vi "CD Init_Prepare Inline Data_Fill Frame Descriptors from BC configuration.vi"(8 "error in (no error)":errorcluster, 11 "RT Channel In":T1 {"RTs"."Mode Codes"."param item refs" format="%.0x"; "RTs"."Mode Codes"."param block data refs"."Data Reference" format="%.0x"; "RTs"."Mode Codes"."Timestamp Channel Data Reference" format="%.0x"; "RTs"."subAddresses"."param item refs" format="%.0x"; "RTs"."subAddresses"."param blocj data refs"."Data Reference" format="%.0x"; "RTs"."subAddresses"."Timestamp Channel Data Reference" format="%.0x"; "RTs"."Status Channel Data Reference" format="%.0x"; "RTs"."Command Channels Refs" format="%.0x"; "BC"."Acyclic Frames Trigger Channels Refs" format="%.0x"; "BC"."Command Channels Refs" format="%.0x"; "BC"."messages"."Timestamp Channel Data Reference" format="%.0x"; "BC"."messages"."Status Channel Data Refs" format="%.0x"; "BC"."messages"."param item refs" format="%.0x"; "BC"."messages"."param Block Data Refs"."Data Reference" format="%.0x"}) -> (0 "error out":errorcluster, 2 "RTs":T13[](array[typedef]) {"Mode Codes"."param item refs" format="%.0x"; "Mode Codes"."param block data refs"."Data Reference" format="%.0x"; "Mode Codes"."Timestamp Channel Data Reference" format="%.0x"; "subAddresses"."param item refs" format="%.0x"; "subAddresses"."param blocj data refs"."Data Reference" format="%.0x"; "subAddresses"."Timestamp Channel Data Reference" format="%.0x"; "Status Channel Data Reference" format="%.0x"; "Command Channels Refs" format="%.0x"}, 3 "Frames Descriptors Out":T18[](array[typedef]) {"RT"."Status Channel Ref" format="%.0x"; "RT"."Words Block Data Refs"."Data Reference" format="%.0x"; "RT"."Timestamp Channel Data Reference" format="%.0x"; "BC"."Status Channel Refs" format="%.0x"; "BC"."param block data refs"."Data Reference" format="%.0x"; "BC"."Timestamp Channel Data Reference" format="%.0x"})   [LabVIEW 2020, in "Ballard MIL-1553 Engine.lvlib"]
uses:
  Ballard MIL-1553 Engine.lvlib
  Controls/RT Inline Frame Descriptor.ctl
  Controls/RT Inline Frame Descriptor_BC.ctl
  <vilib>/NI VeriStand/Custom Device API/Data Reference.ctl
  <vilib>/NI VeriStand/Custom Device API/Block Data Reference.ctl
  <vilib>/NI VeriStand/Custom Device API/Custom Device Item Ref.ctl
  Shared/EncodeDecode/_typedefs/parameter_config_type.ctl
  Shared/EncodeDecode/_typedefs/parameter_config_type_type.ctl
  Shared/EncodeDecode/_typedefs/parameter_config_encoding_type.ctl
  Controls/RT Inline Frame Descriptor_RT.ctl
  Shared/Controls and Global/RT CWD2.ctl
  Shared/Controls and Global/RT CWD1.ctl
  Shared/Controls and Global/RT messageType.ctl
  Shared/Controls and Global/RT Remote Terminal.ctl
  Shared/Controls and Global/RT Remote Terminal_rtMode.ctl
  Shared/Controls and Global/RT Remote Terminal_RT subAddress.ctl
  Shared/Controls and Global/RT Remote Terminal_RT direction.ctl
  Shared/Controls and Global/RT Remote Terminal_RT Mode Code.ctl
  Shared/Controls and Global/RT Channel.ctl
  Shared/Controls and Global/RT BC.ctl
  Shared/Controls and Global/RT Message.ctl
  Shared/Ballard 1553 Shared.lvlib
  <vilib>/NI VeriStand/Custom Device API/Custom Device API.lvlib
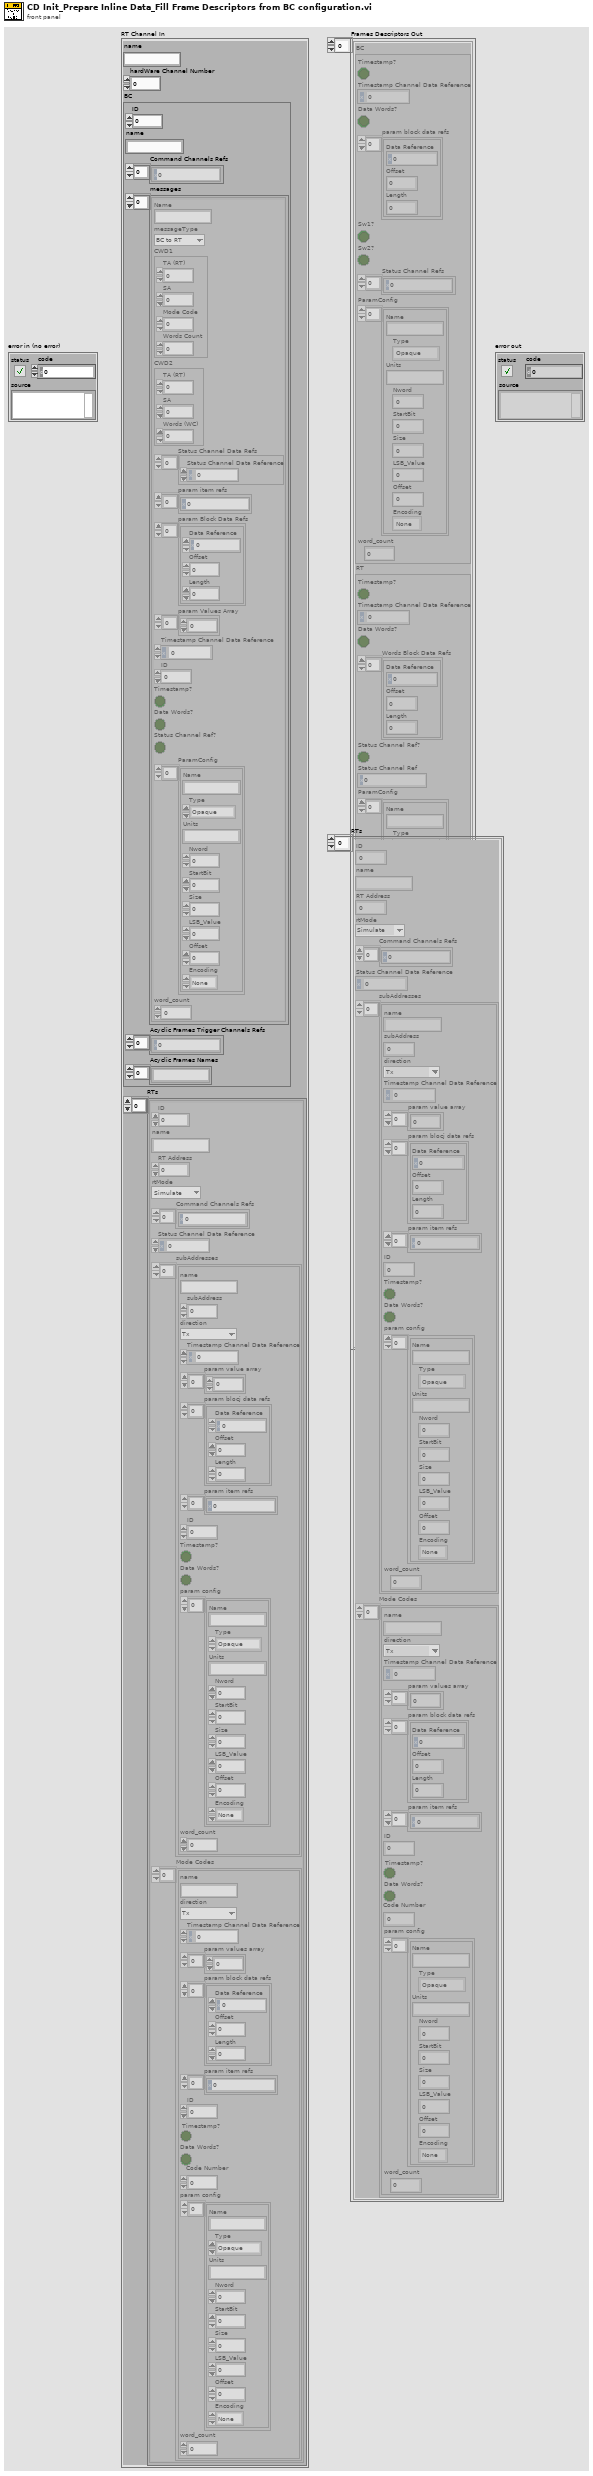
[diagram p1: front panel]
types:
  T1 = typedef "Ballard 1553 Shared.lvlib/RT Channel.ctl" = cluster{"name":string, "hardWare Channel Number":u16, "BC":T2, "RTs":T13[]}
  T2 = typedef "Ballard 1553 Shared.lvlib/RT BC.ctl" = cluster{"ID":i32, "name":string, "Command Channels Refs":T3[], "messages":T4[], "Acyclic Frames Trigger Channels Refs":T3[], "Acyclic Frames Names":string[]}
  T3 = typedef "Custom Device API.lvlib/Custom Device Item Ref.ctl" = u64
  T4 = typedef "Ballard 1553 Shared.lvlib/RT Message.ctl" = cluster{"Name":string, "messageType":T5, "CWD1":T6, "CWD2":T7, "Status Channel Data Refs":T8[], "param item refs":T3[], "param Block Data Refs":T9[], "param Values Array":u16[], "Timestamp Channel Data Reference":T8, "ID":i32, "Timestamp?":bool, "Data Words?":bool, "Status Channel Ref?":bool, "ParamConfig":T10[], "word_count":u8}
  T5 = typedef "Ballard 1553 Shared.lvlib/RT messageType.ctl" = enum16{"BC to RT", "RT to BC", "RT to RT", "MC (Rx)", "MC (Tx)"}
  T6 = typedef "Ballard 1553 Shared.lvlib/RT CWD1.ctl" = cluster{"TA (RT)":i8, "SA":i8, "Mode Code":i8, "Words Count":i8}
  T7 = typedef "Ballard 1553 Shared.lvlib/RT CWD2.ctl" = cluster{"TA (RT)":i8, "SA":i8, "Words (WC)":i8}
  T8 = typedef "Custom Device API.lvlib/Data Reference.ctl" = i32
  T9 = typedef "Custom Device API.lvlib/Block Data Reference.ctl" = cluster{"Data Reference":T8, "Offset":u64, "Length":u64}
  T10 = typedef "parameter_config_type.ctl" = cluster{"Name":string, "Type":T11, "Units":string, "Nword":i32, "StartBit":i32, "Size":i32, "LSB_Value":i32, "Offset":i32, "Encoding":T12}
  T11 = typedef "parameter_config_type_type.ctl" = enum16{"Opaque", "Enum", "Float", "Integer", "Bcd", "Bool"}
  T12 = typedef "parameter_config_encoding_type.ctl" = enum16{"None", "2-complement", "Unsigned"}
  T13 = typedef "Ballard 1553 Shared.lvlib/RT Remote Terminal.ctl" = cluster{"ID":i32, "name":string, "RT Address":i32, "rtMode":T14, "Command Channels Refs":T3[], "Status Channel Data Reference":T8, "subAddresses":T15[], "Mode Codes":T17[]}
  T14 = typedef "Ballard 1553 Shared.lvlib/RT Remote Terminal_rtMode.ctl" = enum16{"Simulate", "Monitor", "Disable"}
  T15 = typedef "Ballard 1553 Shared.lvlib/RT Remote Terminal_RT subAddress.ctl" = cluster{"name":string, "subAddress":i8, "direction":T16, "Timestamp Channel Data Reference":T8, "param value array":u16[], "param blocj data refs":T9[], "param item refs":T3[], "ID":i32, "Timestamp?":bool, "Data Words?":bool, "param config":T10[], "word_count":u8}
  T16 = typedef "Ballard 1553 Shared.lvlib/RT Remote Terminal_RT direction.ctl" = enum16{"Tx", "Rx"}
  T17 = typedef "Ballard 1553 Shared.lvlib/RT Remote Terminal_RT Mode Code.ctl" = cluster{"name":string, "direction":T16, "Timestamp Channel Data Reference":T8, "param values array":u16[], "param block data refs":T9[], "param item refs":T3[], "ID":i32, "Timestamp?":bool, "Data Words?":bool, "Code Number":i32, "param config":T10[], "word_count":u8}
  T18 = typedef "Ballard MIL-1553 Engine.lvlib/RT Inline Frame Descriptor.ctl" = cluster{"BC":T19, "RT":T20, "Initialized?":bool, "RT to RT?":bool, "CWD2":T7, "CWD1":T6, "messageType":T5, "Name":string}
  T19 = typedef "Ballard MIL-1553 Engine.lvlib/RT Inline Frame Descriptor_BC.ctl" = cluster{"Timestamp?":bool, "Timestamp Channel Data Reference":T8, "Data Words?":bool, "param block data refs":T9[], "Sw1?":bool, "Sw2?":bool, "Status Channel Refs":T3[], "ParamConfig":T10[], "word_count":u8}
  T20 = typedef "Ballard MIL-1553 Engine.lvlib/RT Inline Frame Descriptor_RT.ctl" = cluster{"Timestamp?":bool, "Timestamp Channel Data Reference":T8, "Data Words?":bool, "Words Block Data Refs":T9[], "Status Channel Ref?":bool, "Status Channel Ref":T3, "ParamConfig":T10[], "word_count":u8}
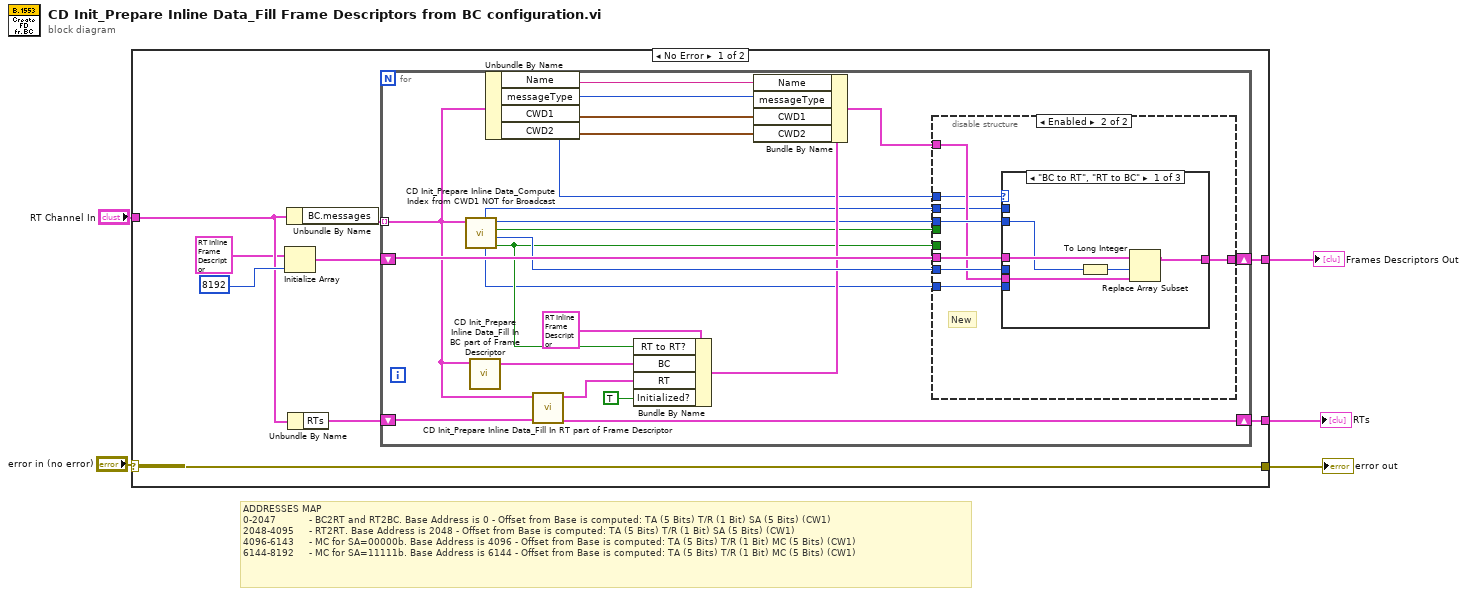
[diagram p0: block diagram]
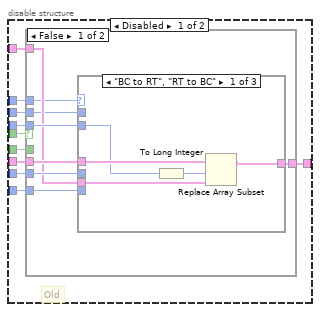
[diagram p2: hidden frame]
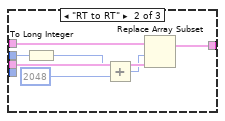
[diagram p3: hidden frame]
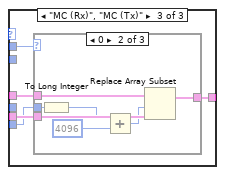
[diagram p4: hidden frame]
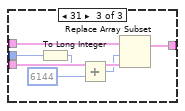
[diagram p6: hidden frame]
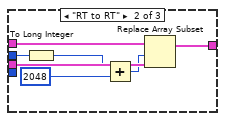
[diagram p8: hidden frame]
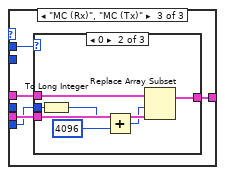
[diagram p9: hidden frame]
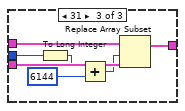
[diagram p11: hidden frame]
diagram:
  # "ADDRESSES MAP \n0-2047           - BC2RT and RT2BC. Base Address is 0 - Offset from Base is computed: TA (5 Bits) T/R (1 Bit) SA (5 Bits) (CW1)\n2048-4095     - RT2RT. Base Address is 2048 - Offset from Base is computed: TA (5 Bits) T/R (1 Bit) SA (5 Bits) (CW1)\n4096-6143     - MC for SA=00000b. Base Address is 4096 - Offset from Base is computed: TA (5 Bits) T/R (1 Bit) MC (5 Bits) (CW1)\n6144-8192     - MC for SA=11111b. Base Address is 6144 - Offset from Base is computed: TA (5 Bits) T/R (1 Bit) MC (5 Bits) (CW1)"
  n1 = case shown="No Error" "error in (no error)" {
    selector: "error in (no error)" -> [w6 w127]
    tunnel: [w13 _] -> w5
    tunnel: [w12 _] -> w4
    tunnel: "RT Channel In" -> [w10 _]
    tunnel: [w6 w127] -> w1
    frame No Error {
      n2 = Initialize Array(T18 {"BC"={"Timestamp?"=FALSE, "Timestamp Channel Data Reference"=0, "Data Words?"=FALSE, "param block data refs"=[], "Sw1?"=FALSE, "Sw2?"=FALSE, "Status Channel Refs"=[], "ParamConfig"=[], "word_count"=0}, "RT"={"Timestamp?"=FALSE, "Timestamp Channel Data Reference"=0, "Data Words?"=FALSE, "Words Block Data Refs"=[], "Status Channel Ref?"=FALSE, "Status Channel Ref"=0, "ParamConfig"=[], "word_count"=0}, "Initialized?"=FALSE, "RT to RT?"=FALSE, "CWD2"={"TA (RT)"=0, "SA"=0, "Words (WC)"=0}, "CWD1"={"TA (RT)"=0, "SA"=0, "Mode Code"=0, "Words Count"=0}, "messageType"=enum."BC to RT", "Name"=""} ("Frame Descriptor"), 8192 ("dimension size")) -> (w8:T18[])
      n3 = Unbundle By Name(w10) -> ("BC.messages"=w9:T4[])
      n4 = Unbundle By Name(w10) -> ("RTs"=w11:T13[])
      n5 = for {
        shift-right: [w34] -> w13
        shift-left: w8 -> [w35]
        tunnel: w9 -> [w22] mode=indexing
        shift-right: [w19] -> w12
        shift-left: w11 -> [w30]
        n6 = call "CD Init_Prepare Inline Data_Compute Index from CWD1 NOT for Broadcast.vi"("message"=w22) -> ("RT to RT?"=w20:bool, "Index 1"=w28:u32, "Broadcast?"=w18:bool, "Index 0"=w23:u16, "Index 2"=w16:u16, "CWD1.SA"=w15:i8)  [unwired: 5 in]
        n7 = call "CD Init_Prepare Inline Data_Fill In BC part of Frame Descriptor.vi"("message"=w22) -> ("BC Frame Descriptor"=w32:T19)  [unwired: 10 in]
        n8 = Unbundle By Name(w22) -> ("Name"=w26:string, "messageType"=w17:T5, "CWD1"=w25:T6, "CWD2"=w24:T7)
        n9 = call "CD Init_Prepare Inline Data_Fill In RT part of Frame Descriptor.vi"("RTs In"=w30, "message"=w22) -> ("RTs Out"=w19:T13[], "RT Frame Descriptor"=w31:T20)  [unwired: 8 in]
        n10 = Bundle By Name(cluster=T18 {"BC"={"Timestamp?"=FALSE, "Timestamp Channel Data Reference"=0, "Data Words?"=FALSE, "param block data refs"=[], "Sw1?"=FALSE, "Sw2?"=FALSE, "Status Channel Refs"=[], "ParamConfig"=[], "word_count"=0}, "RT"={"Timestamp?"=FALSE, "Timestamp Channel Data Reference"=0, "Data Words?"=FALSE, "Words Block Data Refs"=[], "Status Channel Ref?"=FALSE, "Status Channel Ref"=0, "ParamConfig"=[], "word_count"=0}, "Initialized?"=FALSE, "RT to RT?"=FALSE, "CWD2"={"TA (RT)"=0, "SA"=0, "Words (WC)"=0}, "CWD1"={"TA (RT)"=0, "SA"=0, "Mode Code"=0, "Words Count"=0}, "messageType"=enum."BC to RT", "Name"=""} ("Frame Descriptor"), "RT to RT?"=w20, "BC"=w32, "RT"=w31, "Initialized?"=TRUE) -> (w27:T18)
        n11 = Bundle By Name(cluster=w27, "Name"=w26, "messageType"=w17, "CWD1"=w25, "CWD2"=w24) -> (w21:T18)
        n12 = disable-structure shown="Enabled" {
          disable-tunnel: w35 -> [w45 w94]
          disable-tunnel: [w44 w93] -> w34
          disable-tunnel: w28 -> [w43 w92]
          disable-tunnel: w23 -> [w42 w91]
          disable-tunnel: w21 -> [w41 w90]
          disable-tunnel: w20 -> [w40 _]
          disable-tunnel: w18 -> [w39 _]
          disable-tunnel: w17 -> [w38 w89]
          disable-tunnel: w16 -> [w37 w88]
          disable-tunnel: w15 -> [w36 w87]
          frame Disabled {
            # "Old"
            n13 = case shown="False" w39 {
              tunnel: w45 -> [w53 w86]
              tunnel: [w52 w86] -> w44
              tunnel: w43 -> [w51 _]
              tunnel: w42 -> [w50 _]
              tunnel: w41 -> [w49 _]
              tunnel: w40 -> [_ _]
              tunnel: w38 -> [w48 _]
              tunnel: w37 -> [w46 _]
              tunnel: w36 -> [w47 _]
              frame False {
                n14 = case shown="\"BC to RT\", \"RT to BC\"" w48 {
                  tunnel: w53 -> [w58 w65 w70]
                  tunnel: [w57 w64 w69] -> w52
                  tunnel: w51 -> [_ w60 _]
                  tunnel: w49 -> [w55 w63 w68]
                  tunnel: w50 -> [w54 _ _]
                  tunnel: w47 -> [_ _ w67]
                  tunnel: w46 -> [_ _ w66]
                  frame "BC to RT", "RT to BC" {
                    n15 = To Long Integer(number=w54) -> (32bit integer=w56:i32)
                    n16 = Replace Array Subset(array=w58, new element=w55, index=w56) -> (w57:T18[])
                  }
                  frame "RT to RT" {
                    n17 = To Long Integer(number=w60) -> (32bit integer=w62:i32)
                    n18 = Add(x=w62, y=2048) -> (x+y=w61:i32)
                    n19 = Replace Array Subset(array=w65, new element=w63, index=w61) -> (w64:T18[])
                  }
                  frame "MC (Rx)", "MC (Tx)" {
                    n20 = case shown="0" w67 {
                      tunnel: w70 -> [w71 w78 w85]
                      tunnel: [w71 w77 w84] -> w69
                      tunnel: w68 -> [_ w76 w83]
                      tunnel: w66 -> [_ w73 w80]
                      frame 1, Default {
                      }
                      frame 0 {
                        n21 = To Long Integer(number=w73) -> (32bit integer=w75:i32)
                        n22 = Add(x=w75, y=4096) -> (x+y=w74:i32)
                        n23 = Replace Array Subset(array=w78, new element=w76, index=w74) -> (w77:T18[])
                      }
                      frame 31 {
                        n24 = To Long Integer(number=w80) -> (32bit integer=w82:i32)
                        n25 = Add(x=w82, y=6144) -> (x+y=w81:i32)
                        n26 = Replace Array Subset(array=w85, new element=w83, index=w81) -> (w84:T18[])
                      }
                    }
                  }
                }
              }
              frame True {
              }
            }
          }
          frame Enabled {
            # "New"
            n27 = case shown="\"BC to RT\", \"RT to BC\"" w89 {
              tunnel: w94 -> [w99 w106 w111]
              tunnel: [w98 w105 w110] -> w93
              tunnel: w92 -> [_ w101 _]
              tunnel: w90 -> [w96 w104 w109]
              tunnel: w91 -> [w95 _ _]
              tunnel: w87 -> [_ _ w108]
              tunnel: w88 -> [_ _ w107]
              frame "BC to RT", "RT to BC" {
                n28 = To Long Integer(number=w95) -> (32bit integer=w97:i32)
                n29 = Replace Array Subset(array=w99, new element=w96, index=w97) -> (w98:T18[])
              }
              frame "RT to RT" {
                n30 = To Long Integer(number=w101) -> (32bit integer=w103:i32)
                n31 = Add(x=w103, y=2048) -> (x+y=w102:i32)
                n32 = Replace Array Subset(array=w106, new element=w104, index=w102) -> (w105:T18[])
              }
              frame "MC (Rx)", "MC (Tx)" {
                n33 = case shown="0" w108 {
                  tunnel: w111 -> [w112 w119 w126]
                  tunnel: [w112 w118 w125] -> w110
                  tunnel: w109 -> [_ w117 w124]
                  tunnel: w107 -> [_ w114 w121]
                  frame 1, Default {
                  }
                  frame 0 {
                    n34 = To Long Integer(number=w114) -> (32bit integer=w116:i32)
                    n35 = Add(x=w116, y=4096) -> (x+y=w115:i32)
                    n36 = Replace Array Subset(array=w119, new element=w117, index=w115) -> (w118:T18[])
                  }
                  frame 31 {
                    n37 = To Long Integer(number=w121) -> (32bit integer=w123:i32)
                    n38 = Add(x=w123, y=6144) -> (x+y=w122:i32)
                    n39 = Replace Array Subset(array=w126, new element=w124, index=w122) -> (w125:T18[])
                  }
                }
              }
            }
          }
        }
      }
    }
    frame Error {
    }
  }
  "Frames Descriptors Out" <- w5
  "RTs" <- w4
  "error out" <- w1
